vi "Initialize.vi"(8 "error in (no error)":errorcluster, 9 "Reset (True)":bool=TRUE, 10 "ID Query (True)":bool=TRUE, 11 "VISA resource name":refnum<visa-resource-name>) -> (0 "error out":errorcluster, 3 "VISA resource name out":refnum<visa-resource-name>)   [LabVIEW 2014, in "Agilent ESA PSA Series.lvlib"]
doc: "Establishes communication with the instrument and optionally performs an instrument identification query and/or an instrument reset. It also places the instrument in a default state needed for other instrument driver operations. Therefore, call this VI before calling other instrument driver VIs for this instrument. Generally, you need to call the Initialize VI only once at the beginning of an application."
uses:
  Agilent ESA PSA Series.lvlib
  Match Regular Expression.xnode
panel:
  # "(c) 2007-2015 National Instruments.  ALL RIGHTS RESERVED."
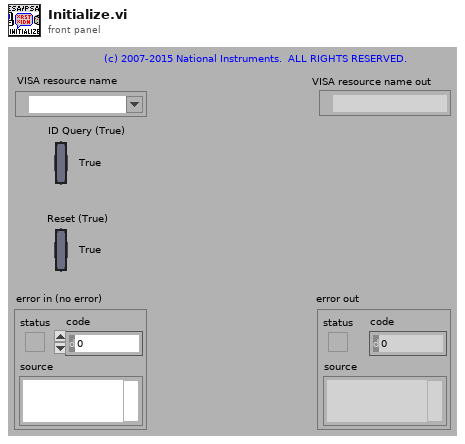
[diagram p1: front panel]
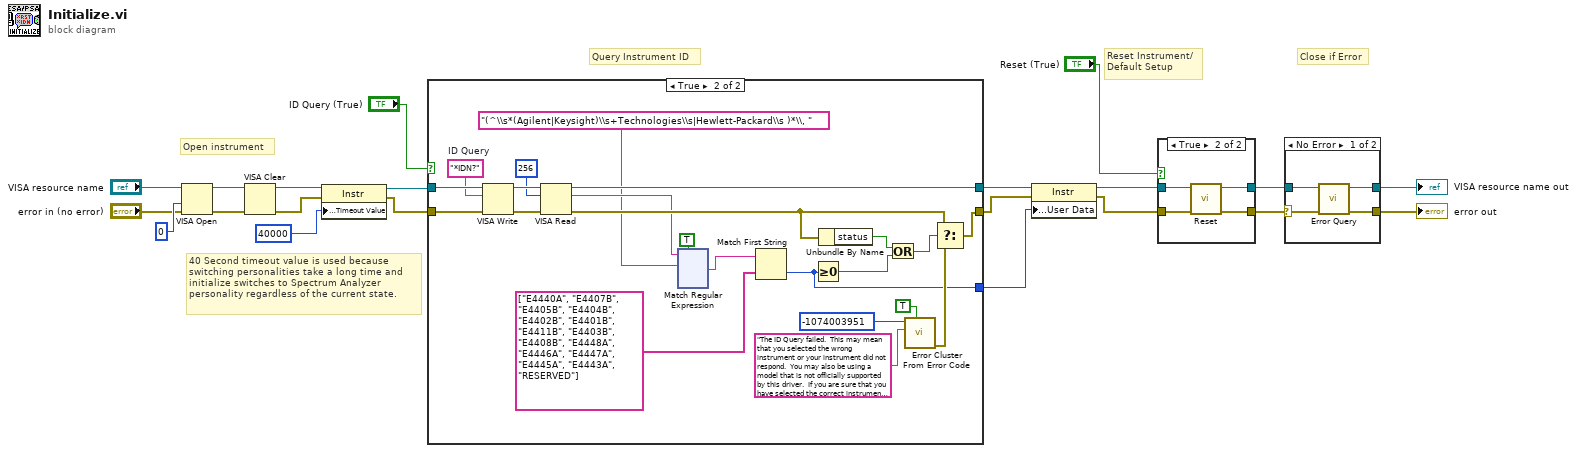
[diagram p0: block diagram]
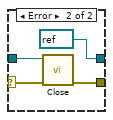
[diagram p2: hidden frame]
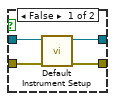
[diagram p3: hidden frame]
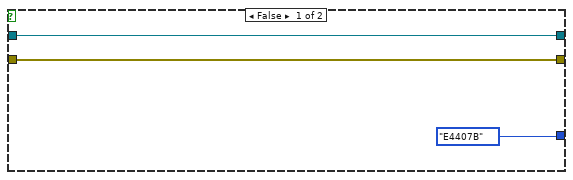
[diagram p4: hidden frame]
diagram:
  # "40 Second timeout value is used because\nswitching personalities take a long time and\ninitialize switches to Spectrum Analyzer\npersonality regardless of the current state."
  # "Close if Error"
  # "Query Instrument ID"
  # "Reset Instrument/\nDefault Setup"
  # "Open instrument"
  n1 = VISA Open(access mode=u32 0, error in (no error)="error in (no error)", VISA resource name="VISA resource name") -> (VISA resource name=w18:refnum<visa-resource-name>, error out=w17:errorcluster)  [unwired: 2 in]
  n2 = VISA Clear(VISA resource name=w18, error in (no error)=w17) -> (VISA resource name out=w4:refnum<visa-resource-name>, error out=w3:errorcluster)
  n3 = property on="Property Node" class="Instr"(reference=w4, error in=w3, "General Settings:Timeout Value"=u32 40000) -> (reference out=w2:refnum<visa-resource-name>, error out=w1:errorcluster)
  n4 = case shown="True" "ID Query (True)" {
    tunnel: [w23 w46] -> w10
    tunnel: [w24 w43] -> w12
    tunnel: w2 -> [w24 w44]
    tunnel: w1 -> [w23 w45]
    tunnel: [enum16{"E4407B"}."E4407B" w30] -> w8
    frame False {
    }
    frame True {
      w39 = "*IDN?"  # ID Query
      n5 = VISA Write(VISA resource name=w44, write buffer=w39, error in (no error)=w45) -> (VISA resource name out=w42:refnum<visa-resource-name>, error out=w41:errorcluster)  [unwired: 1 out]
      n6 = VISA Read(VISA resource name=w42, byte count=u32 256, error in (no error)=w41) -> (VISA resource name out=w43:refnum<visa-resource-name>, read buffer=w27:string, error out=w34:errorcluster)  [unwired: 1 out]
      n7 = xnode ("Match Regular Expression")("input string"=w27, "regular expression"="(^\\s*(Agilent|Keysight)\\s+Technologies\\s|Hewlett-Packard\\s )*\\, " ("Company Name Regular Expression"), "ignore case? (F)"=TRUE) -> ("after match"=w25:string)  [unwired: 3 in, 4 out]
      n8 = Match First String(2:string[] ["E4440A", "E4407B", "E4405B", "E4404B", "E4402B", "E4401B", "E4411B", "E4403B", "E4408B", "E4448A", "E4446A", "E4447A", "E4445A", "E4443A", "RESERVED"], 3:w25) -> (0:w30:i32)  [unwired: 1 out]
      n9 = Greater Or Equal To 0?(x=w30) -> (x >= 0?=w32:bool)
      n10 = Unbundle By Name(w34) -> ("status"=w33:bool)
      n11 = Or(x=w33, y=w32) -> (x .or. y?=w31:bool)
      n12 = call "Error Cluster From Error Code.vi"("show call chain? (False)"=TRUE, "error message (\"\")"="The ID Query failed.  This may mean that you selected the wrong instrument or your instrument did not respond.  You may also be using a model that is not officially supported by this driver.  If you are sure that you have selected the correct instrument and it is responding, try disabling the ID Query." ("Source (VI Name)"), "error code (0)"=-1074003951 ("Code")) -> ("error out"=w38:errorcluster)  [unwired: 6 in]
      n13 = Select(t=w34, s=w31, f=w38) -> (s? t:f=w46:errorcluster)
    }
  }
  n14 = property class="Instr"(reference=w12, error in=w10, "General Settings:User Data"=w8) -> (reference out=w11:refnum<visa-resource-name>, error out=w9:errorcluster)
  n15 = case shown="True" "Reset (True)" {
    tunnel: w9 -> [w163 w165]
    tunnel: [w162 w168] -> w13
    tunnel: w11 -> [w164 w166]
    tunnel: [w161 w167] -> w14
    frame False {
      n16 = call "Default Instrument Setup.vi"("error in (no error)"=w163, "VISA resource name"=w164) -> ("error out"=w162:errorcluster, "VISA resource name out"=w161:refnum<visa-resource-name>)  [unwired: 8 in]
    }
    frame True {
      n17 = call "Reset.vi"("error in (no error)"=w165, "VISA resource name"=w166) -> ("error out"=w168:errorcluster, "VISA resource name out"=w167:refnum<visa-resource-name>)  [unwired: 8 in]
    }
  }
  n18 = case shown="No Error" w13 {
    selector: w13 -> [w170 w174]
    tunnel: w14 -> [w169 w175]
    tunnel: [w172 refnum<visa-resource-name> refnum ("VISA resource name out")] -> w16
    tunnel: [w171 w176] -> w15
    frame No Error {
      n19 = call "Error Query.vi"("error in (no error)"=w170, "VISA resource name"=w169) -> ("error out"=w171:errorcluster, "VISA resource name out"=w172:refnum<visa-resource-name>)  [unwired: 6 in, 2 out]
    }
    frame Error {
      n20 = call "Close.vi"("error in (no error)"=w174, "VISA resource name"=w175) -> ("error out"=w176:errorcluster)  [unwired: 9 in]
    }
  }
  "VISA resource name out" <- w16
  "error out" <- w15
